vi "HV_Status_to_Bool.vi"(8 "Column":i32, 9 "False":string, 10 "True":string, 11 "Status Array":string[][](array[string])) -> (3 "Array":bool[](array[boolean]))   [LabVIEW 2018]
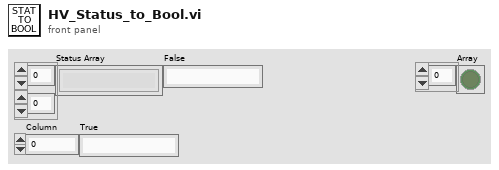
[diagram p1: front panel]
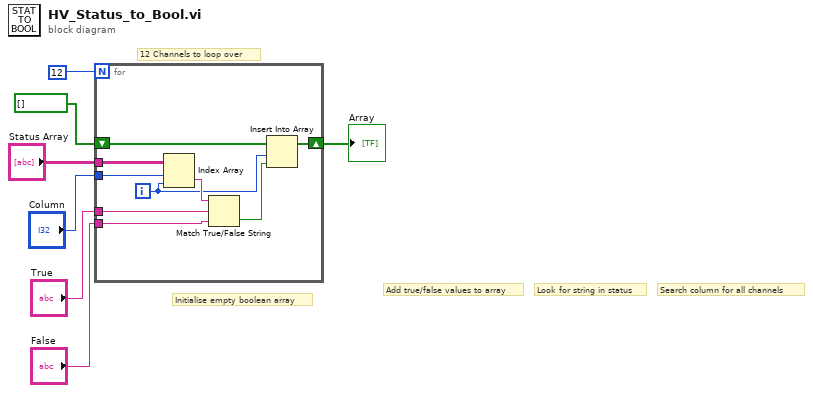
[diagram p0: block diagram]
diagram:
  # "Add true/false values to array"
  # "Initialise empty boolean array"
  # "12 Channels to loop over"
  # "Look for string in status"
  # "Search column for all channels"
  n1 = for {
    N: 12 -> [_]
    tunnel: "Status Array" -> [w16]
    tunnel: "Column" -> [w14]
    tunnel: "True" -> [w13]
    tunnel: "False" -> [w12]
    shift-right: [w8] -> w1
    shift-left: bool[] [] -> [w9]
    i -> [w10]
    n2 = Index Array "Index Array"(array=w16, index (row)=w14, index (col)=w10) -> (element=w15:string)
    n3 = Match True/False String(2:w12, 3:w13, 4:w15) -> (0:w11:bool)  [unwired: 1 out]
    n4 = Insert Into Array(array=w9, index=w10, new element=w11) -> (w8:bool[])
  }
  "Array" <- w1
